vi "Right Auto V.3.0.vi"(0 "Desired Angle":dbl) -> (7 "Stop":bool)   [LabVIEW 2017]
uses:
  Robot Global Data V.3.0.vi
panel:
  out "Motor Speed":dbl(graph)
  out "Gyro":dbl(graph)
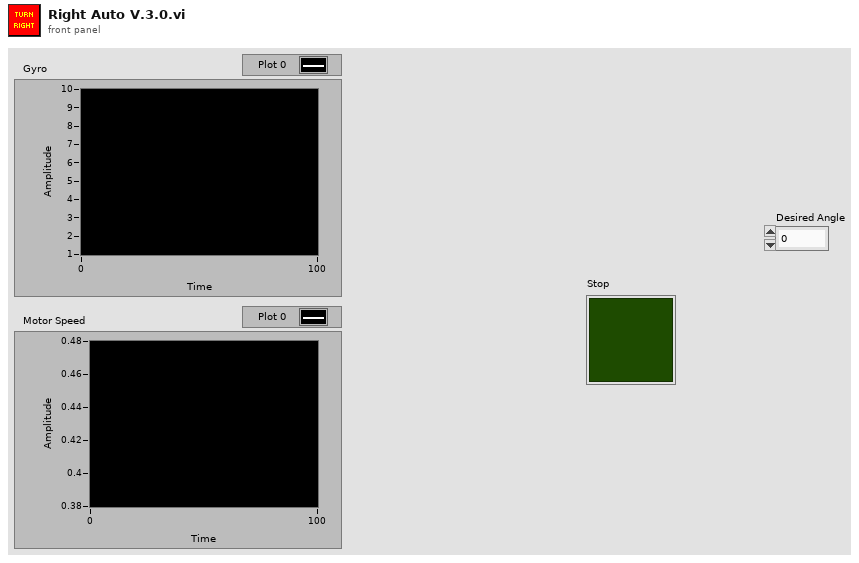
[diagram p1: front panel]
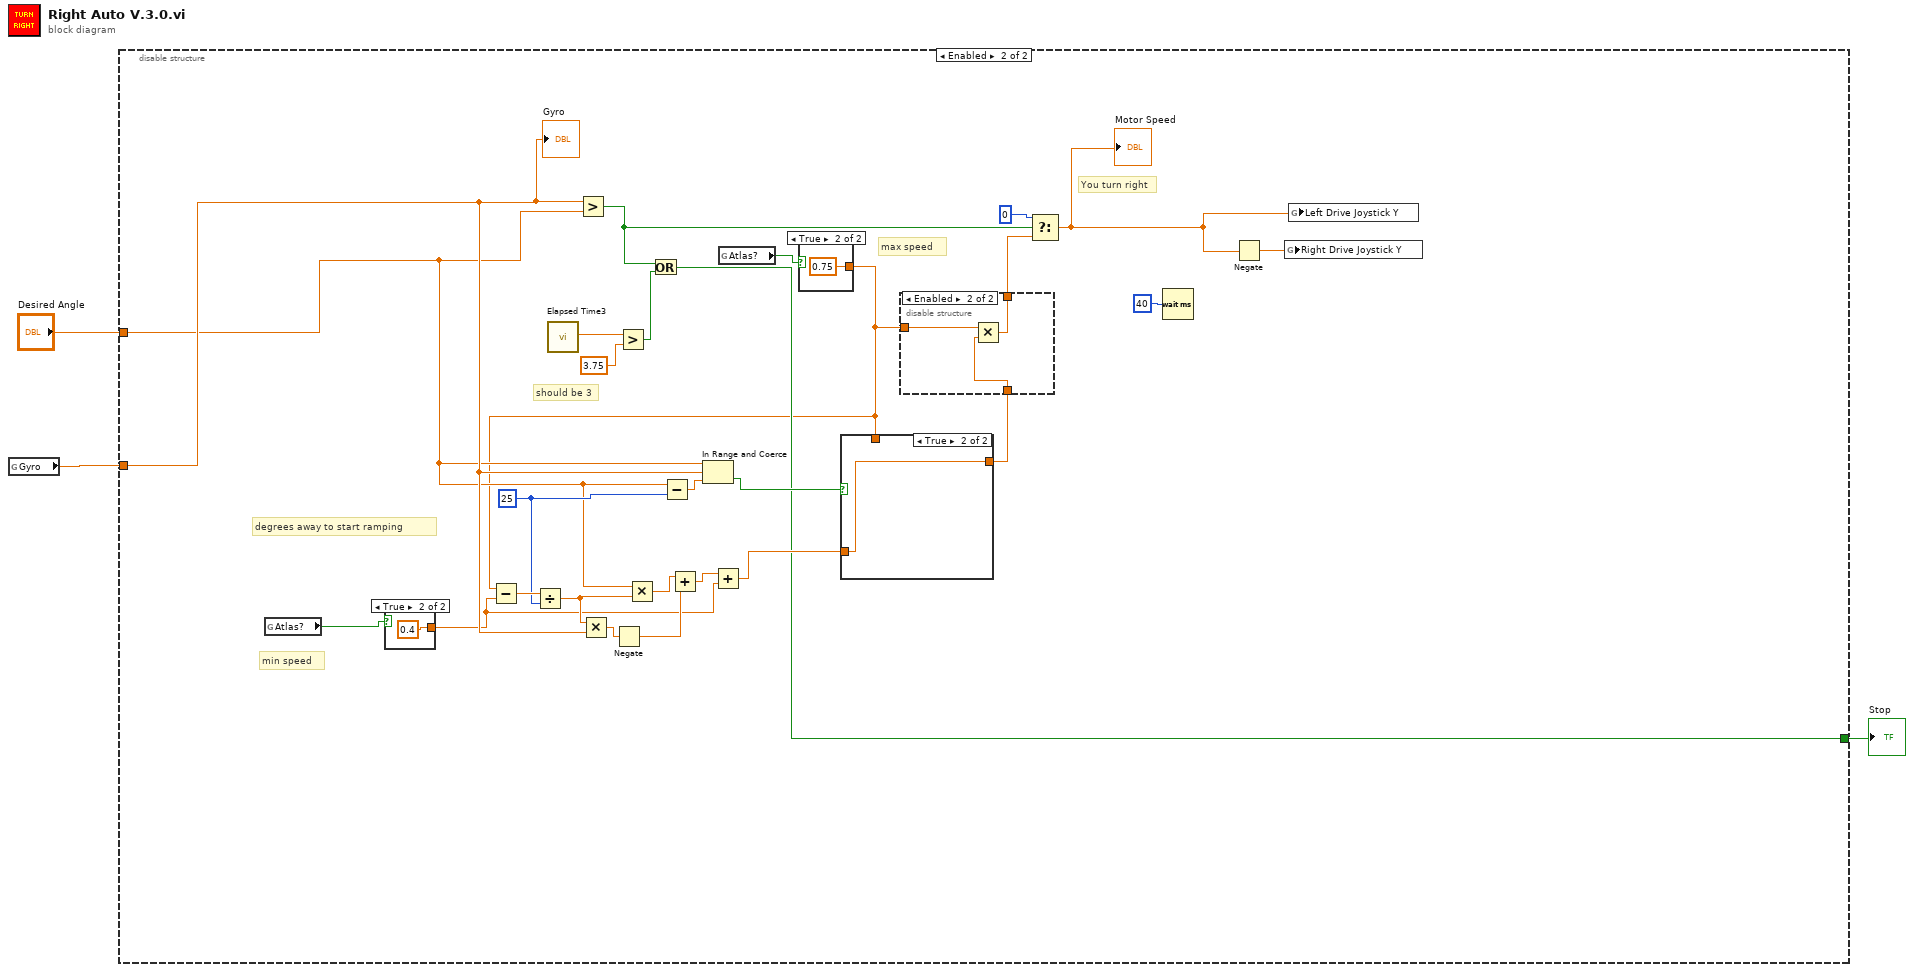
[diagram p0: block diagram]
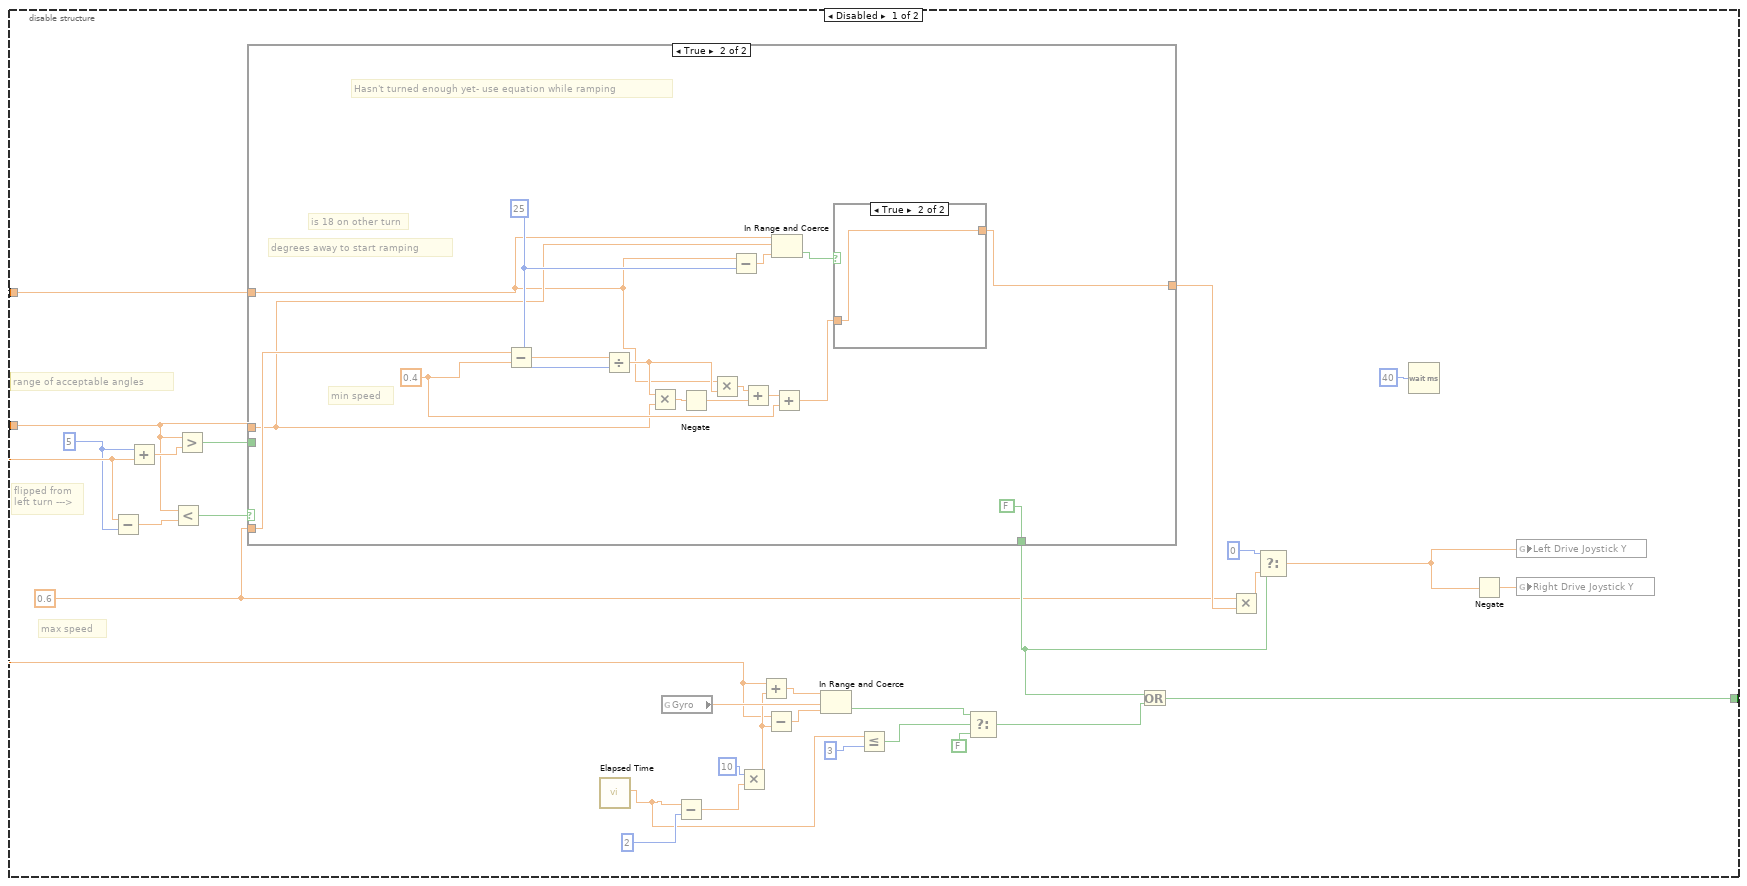
[diagram p2: hidden frame]
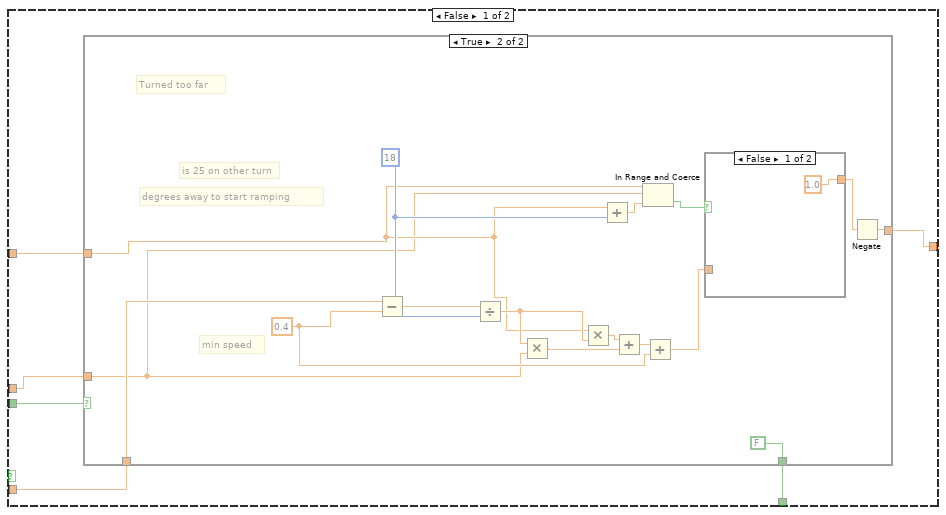
[diagram p3: hidden frame]
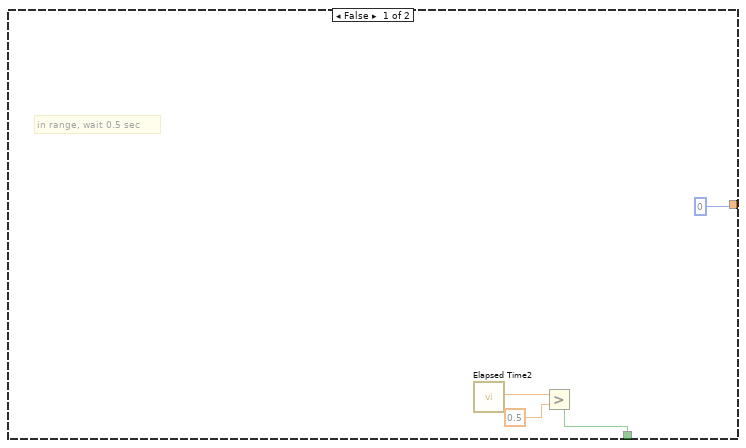
[diagram p4: hidden frame]
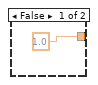
[diagram p6: hidden frame]
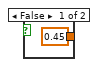
[diagram p7: hidden frame]
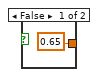
[diagram p8: hidden frame]
diagram:
  n1 = global read "Robot Global Data V.3.0.vi" "Gyro"() -> (w3:dbl)
  n2 = disable-structure shown="Enabled" {
    disable-tunnel: w3 -> [w25 w88]
    disable-tunnel: "Desired Angle" -> [w11 w87]
    disable-tunnel: [w4 w85] -> w1
    frame Disabled {
      w10 = 5
      w5 = 0.6
      # "flipped from\nleft turn --->"
      # "range of acceptable angles"
      # "max speed"
      n3 = Subtract(x=w11, y=w10) -> (x-y=w28:dbl)
      n4 = Add(x=w10, y=w11) -> (x+y=w29:dbl)
      n5 = Less?(x=w25, y=w28) -> (x < y?=w6:bool)
      n6 = Greater?(x=w25, y=w29) -> (0:w7:bool)
      n7 = case shown="True" w6 {
        tunnel: w7 -> [w37 _]
        tunnel: [w38 FALSE] -> w27
        tunnel: w25 -> [w33 w62]
        tunnel: w5 -> [w34 w64]
        tunnel: w11 -> [w35 w61]
        tunnel: [w36 w63] -> w26
        frame False {
          n8 = case shown="True" w37 {
            tunnel: [w40 FALSE] -> w38
            tunnel: [0 w44] -> w36
            tunnel: w35 -> [_ w48]
            tunnel: w34 -> [_ w47]
            tunnel: w33 -> [_ w46]
            frame False {
              # "in range, wait 0.5 sec"
              n9 = call "Elapsed Time2"() -> ("Elapsed Time (s)"=w42:dbl)  [unwired: 12 in, 7 out]
              n10 = Greater?(x=w42, y=0.5) -> (0:w40:bool)
            }
            frame True {
              w50 = 18
              w49 = 0.4
              # "is 25 on other turn"
              # "degrees away to start ramping"
              # "min speed"
              # "Turned too far"
              n11 = Subtract(x=w47, y=w49) -> (x-y=w56:dbl)
              n12 = Divide(x=w56, y=w50) -> (x/y=w57:dbl)
              n13 = Multiply(x=w57, y=w46) -> (x*y=w45:dbl)
              n14 = Multiply(x=w48, y=w57) -> (x*y=w53:dbl)
              n15 = Add(x=w48, y=w50) -> (x+y=w51:dbl)
              n16 = Add(x=w53, y=w45) -> (x+y=w54:dbl)
              n17 = In Range and Coerce(upper limit=w48, x=w46, lower limit=w51) -> (In Range?=w52:bool)  [unwired: 1 out]
              n18 = Add(x=w54, y=w49) -> (x+y=w55:dbl)
              n19 = case shown="False" w52 {
                tunnel: w55 -> [_ w60]
                tunnel: [1.0 w60] -> w43
                frame False {
                }
                frame True {
                }
              }
              n20 = Negate(x=w43) -> (-x=w44:dbl)
            }
          }
        }
        frame True {
          w66 = 25
          w65 = 0.4
          # "is 18 on other turn"
          # "degrees away to start ramping"
          # "min speed"
          # "Hasn't turned enough yet- use equation while ramping"
          n21 = Subtract(x=w64, y=w65) -> (x-y=w74:dbl)
          n22 = Divide(x=w74, y=w66) -> (x/y=w75:dbl)
          n23 = Multiply(x=w75, y=w62) -> (x*y=w69:dbl)
          n24 = Negate(x=w69) -> (-x=w71:dbl)
          n25 = Multiply(x=w61, y=w75) -> (x*y=w70:dbl)
          n26 = Subtract(x=w61, y=w66) -> (x-y=w67:dbl)
          n27 = Add(x=w70, y=w71) -> (x+y=w72:dbl)
          n28 = In Range and Coerce(upper limit=w61, x=w62, lower limit=w67) -> (In Range?=w68:bool)  [unwired: 1 out]
          n29 = Add(x=w72, y=w65) -> (x+y=w73:dbl)
          n30 = case shown="True" w68 {
            tunnel: w73 -> [_ w78]
            tunnel: [1.0 w78] -> w63
            frame False {
            }
            frame True {
            }
          }
        }
      }
      n31 = call "Elapsed Time"() -> ("Elapsed Time (s)"=w17:dbl)  [unwired: 12 in, 7 out]
      n32 = global read "Robot Global Data V.3.0.vi" "Gyro"() -> (w22:dbl)
      n33 = Subtract(x=w17, y=2) -> (x-y=w19:dbl)
      n34 = Multiply(x=10, y=w19) -> (x*y=w18:dbl)
      n35 = Add(x=w11, y=w18) -> (x+y=w24:dbl)
      n36 = Subtract(x=w11, y=w18) -> (x-y=w23:dbl)
      n37 = In Range and Coerce(upper limit=w24, x=w22, lower limit=w23) -> (In Range?=w13:bool)  [unwired: 1 out]
      n38 = Less Or Equal?(x=w17, y=3) -> (x <= y?=w14:bool)
      n39 = Select(t=w13, s=w14, f=FALSE) -> (s? t:f=w15:bool)
      n40 = Or(x=w27, y=w15) -> (x .or. y?=w4:bool)
      n41 = Multiply(x=w5, y=w26) -> (x*y=w30:dbl)
      n42 = Select(t=0, s=w27, f=w30) -> (s? t:f=w8:dbl)
      n43 = Wait (ms)(milliseconds to wait=u32 40) -> ()  [unwired: 1 out]
      n44 = Negate(x=w8) -> (-x=w9:dbl)
      n45 = global write "Robot Global Data V.3.0.vi" "Left Drive Joystick Y"(w8) -> ()
      n46 = global write "Robot Global Data V.3.0.vi" "Right Drive Joystick Y"(w9) -> ()
    }
    frame Enabled {
      w95 = 25
      # "min speed"
      # "should be 3"
      # "degrees away to start ramping"
      # "max speed"
      # "You turn right"
      n47 = global read "Robot Global Data V.3.0.vi" "Atlas?"() -> (w80:bool)
      n48 = case shown="True" w80 {
        tunnel: [0.45 0.4] -> w79
        frame False {
        }
        frame True {
        }
      }
      n49 = call "Elapsed Time3"() -> ("Elapsed Time (s)"=w92:dbl)  [unwired: 12 in, 7 out]
      n50 = Greater?(x=w88, y=w87) -> (0:w90:bool)
      n51 = Greater?(x=w92, y=3.75) -> (0:w91:bool)
      n52 = Or(x=w90, y=w91) -> (x .or. y?=w85:bool)
      n53 = Subtract(x=w87, y=w95) -> (x-y=w103:dbl)
      n54 = In Range and Coerce(upper limit=w87, x=w88, lower limit=w103) -> (In Range?=w102:bool)  [unwired: 1 out]
      n55 = global read "Robot Global Data V.3.0.vi" "Atlas?"() -> (w81:bool)
      n56 = case shown="True" w81 {
        tunnel: [0.65 0.75] -> w82
        frame False {
        }
        frame True {
        }
      }
      n57 = Subtract(x=w82, y=w79) -> (x-y=w96:dbl)
      n58 = Divide(x=w96, y=w95) -> (x/y=w94:dbl)
      n59 = Multiply(x=w94, y=w88) -> (x*y=w101:dbl)
      n60 = Negate(x=w101) -> (-x=w99:dbl)
      n61 = Multiply(x=w87, y=w94) -> (x*y=w100:dbl)
      n62 = Add(x=w100, y=w99) -> (x+y=w98:dbl)
      n63 = Add(x=w98, y=w79) -> (x+y=w97:dbl)
      n64 = case shown="True" w102 {
        tunnel: w97 -> [_ w115]
        tunnel: [w114 w115] -> w83
        tunnel: w82 -> [w114 _]
        frame False {
        }
        frame True {
        }
      }
      n65 = disable-structure shown="Enabled" {
        disable-tunnel: [w110 w113] -> w84
        disable-tunnel: w83 -> [w110 w112]
        disable-tunnel: w82 -> [_ w111]
        frame Disabled {
        }
        frame Enabled {
          n66 = Multiply(x=w111, y=w112) -> (x*y=w113:dbl)
        }
      }
      n67 = Select(t=0, s=w90, f=w84) -> (s? t:f=w89:dbl)
      "Motor Speed" <- w89
      n68 = Wait (ms)(milliseconds to wait=u32 40) -> ()  [unwired: 1 out]
      n69 = Negate(x=w89) -> (-x=w86:dbl)
      n70 = global write "Robot Global Data V.3.0.vi" "Right Drive Joystick Y"(w86) -> ()
      n71 = global write "Robot Global Data V.3.0.vi" "Left Drive Joystick Y"(w89) -> ()
      "Gyro" <- w88
    }
  }
  "Stop" <- w1
